vi "Server_V2.0.vi"() -> ()   [LabVIEW 2015]
doc: "Creates a named service and listens on the first available port. When a client connects to the service, it sends a response string to the client."
panel:
  in  "Message Type":T1(ring)
  in  "Message to Send":string="You are currently accessing TCP Named Service - Server.vi from client %s on port %d."
  in  "Stop 2":bool
  out "IP":string
  in  "Location Y":string="3"
  in  "Location X":string="3"
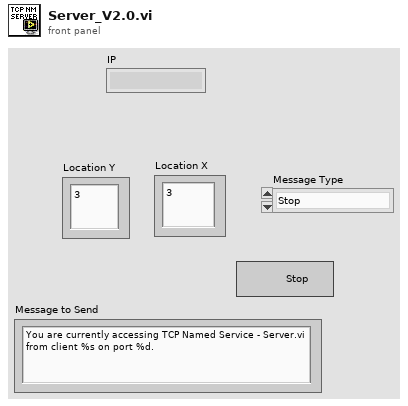
[diagram p1: front panel]
types:
  T1 = enum16{"Stop", "Deploy", "Return to Base", "Location Update", "Recalibrate"}
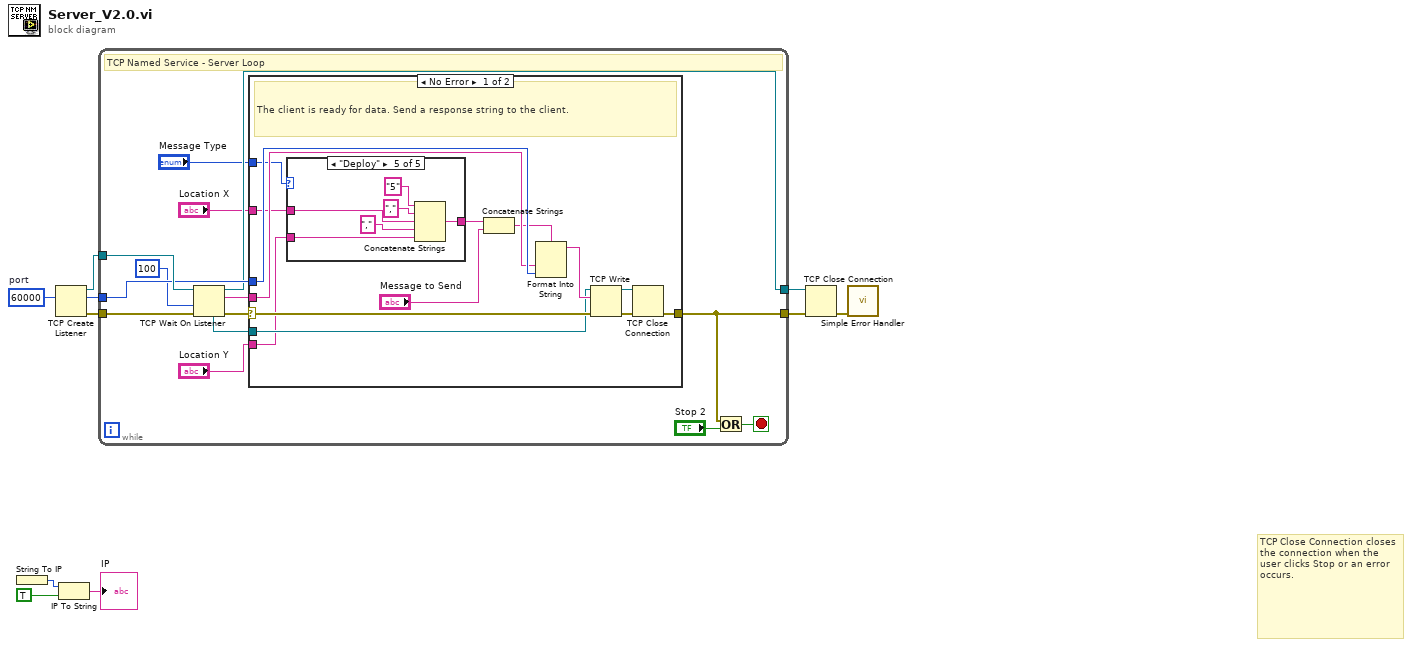
[diagram p0: block diagram]
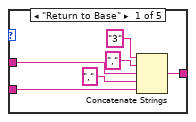
[diagram p2: hidden frame]
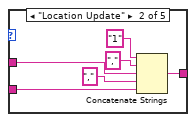
[diagram p3: hidden frame]
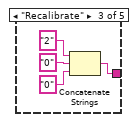
[diagram p4: hidden frame]
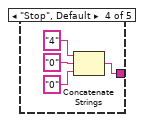
[diagram p5: hidden frame]
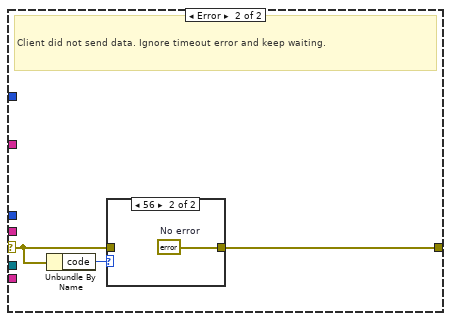
[diagram p6: hidden frame]
diagram:
  w1 = u16 60000  # port
  # "TCP Close Connection closes the connection when the user clicks Stop or an error occurs."
  n1 = String To IP() -> (0:w10:u32)  [unwired: 1 in]
  n2 = TCP Create Listener(10:w1) -> (0:w6:errorcluster, 2:w3:u16, 3:w7:refnum<k5>)  [unwired: 4 in]
  n3 = IP To String(1:TRUE ("dot notation? (F)"), 2:w10) -> (0:→"IP":string)
  n4 = while {
    tunnel: [w17] -> w4
    tunnel: w7 -> [w24]
    tunnel: w6 -> [w22]
    tunnel: [w14] -> w5
    tunnel: w3 -> [w20]
    stop <- w19 stop-if-true
    # "TCP Named Service - Server Loop"
    n5 = TCP Wait On Listener(8:w22, 9:100 ("timeout ms (25000)"), 11:w24) -> (0:w23:errorcluster, 2:w15:string, 3:w14:refnum<k5>, 4:w21:refnum<k5>)  [unwired: 1 in, 1 out]
    n6 = case shown="No Error" w23 {
      selector: w23 -> [w38 w67]
      tunnel: [w32 w65] -> w17
      tunnel: w21 -> [w33 _]
      tunnel: w20 -> [w36 _]
      tunnel: w15 -> [w35 _]
      tunnel: "Message Type" -> [w30 _]
      tunnel: "Location X" -> [w29 _]
      tunnel: "Location Y" -> [w28 _]
      frame No Error {
        # "The client is ready for data. Send a response string to the client."
        n7 = case shown="\"Deploy\"" w30 {
          tunnel: [w39 w50 w51 w55 w59] -> w26
          tunnel: w29 -> [w41 w47 _ _ w61]
          tunnel: w28 -> [w40 w45 _ _ w60]
          frame "Return to Base" {
            n8 = Concatenate Strings("3" ("string"), "," ("string"), w41, "," ("string"), w40) -> (w39:string)
          }
          frame "Location Update" {
            n9 = Concatenate Strings("1" ("string"), "," ("string"), w47, "," ("string"), w45) -> (w50:string)
          }
          frame "Recalibrate" {
            n10 = Concatenate Strings("2" ("string"), "0" ("string"), "0" ("string")) -> (w51:string)
          }
          frame "Stop", Default {
            n11 = Concatenate Strings("4" ("string"), "0" ("string"), "0" ("string")) -> (w55:string)
          }
          frame "Deploy" {
            n12 = Concatenate Strings("5" ("string"), "," ("string"), w61, "," ("string"), w60) -> (w59:string)
          }
        }
        n13 = Concatenate Strings(w26, "Message to Send") -> (w27:string)
        n14 = Format Into String(format string=w27, w35, w36) -> (resulting string=w34:string)  [unwired: 2 in, 1 out]
        n15 = TCP Write(connection ID=w33, data in=w34, error in (no error)=w38) -> (connection ID out=w31:refnum<k5>, error out=w37:errorcluster)  [unwired: 1 in, 1 out]
        n16 = TCP Close Connection(connection ID=w31, error in (no error)=w37) -> (error out=w32:errorcluster)  [unwired: 1 in, 1 out]
      }
      frame Error {
        # "Client did not send data. Ignore timeout error and keep waiting."
        n17 = Unbundle By Name(w67) -> ("code"=w66:i32)
        n18 = case shown="56" w66 {
          tunnel: w67 -> [w68 _]
          tunnel: [w68 w69] -> w65
          frame Default {
          }
          frame 56 {
            w69 = errorcluster {"status"=FALSE, "code"=0, "source"=""}  # No error
          }
        }
      }
    }
    n19 = Or(x=w17, y="Stop 2") -> (x .or. y?=w19:bool)
  }
  n20 = TCP Close Connection(connection ID=w5, error in (no error)=w4) -> (error out=w2:errorcluster)  [unwired: 1 in, 1 out]
  n21 = call <vilib>:"Simple Error Handler.vi"("error in (no error)"=w2) -> ()  [unwired: 4 in, 5 out]
